vi "ConfigureSequencerElement.vi"(4 "error in (no error)":errorcluster, 5 "Sequencer Element":i16=1, 6 "Sequencer Item":T1={"Entry Length"=16384, "Repetition Count"=1, "Infinite Repetitions"=FALSE, "Channels"=[{"Analog Waveform"="SINE", "Amplitude [V]"=2.0, "Offset [V]"=0.0}, {"Analog Waveform"="SINE", "Amplitude [V]"=2.0, "Offset [V]"=0.0}], "Digital Waveform"=""} {"Repetition Count" min=1}, 7 "VISA resource name":refnum<visa-resource-name>) -> (0 "error out":errorcluster, 3 "VISA resource name out":refnum<visa-resource-name>)   [LabVIEW 2020, in "Active Technologies AWG3000.lvlib"]
uses:
  Active Technologies AWG3000.lvlib
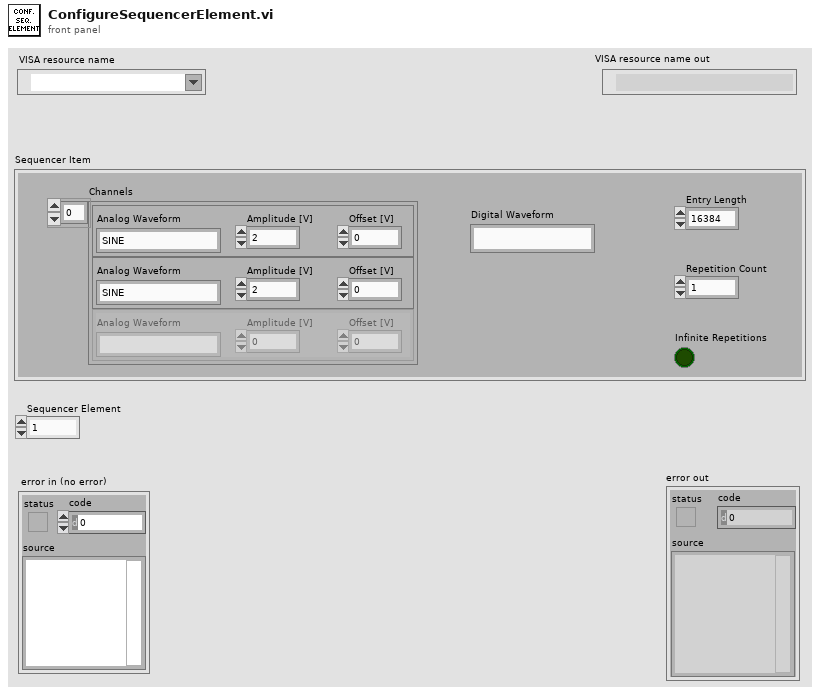
[diagram p1: front panel]
types:
  T1 = cluster{"Entry Length":i32, "Repetition Count":i32, "Infinite Repetitions":bool, "Channels":cluster{"Analog Waveform":string, "Amplitude [V]":dbl, "Offset [V]":dbl}[], "Digital Waveform":string}
  T2 = cluster{"Analog Waveform":string, "Amplitude [V]":dbl, "Offset [V]":dbl}[]
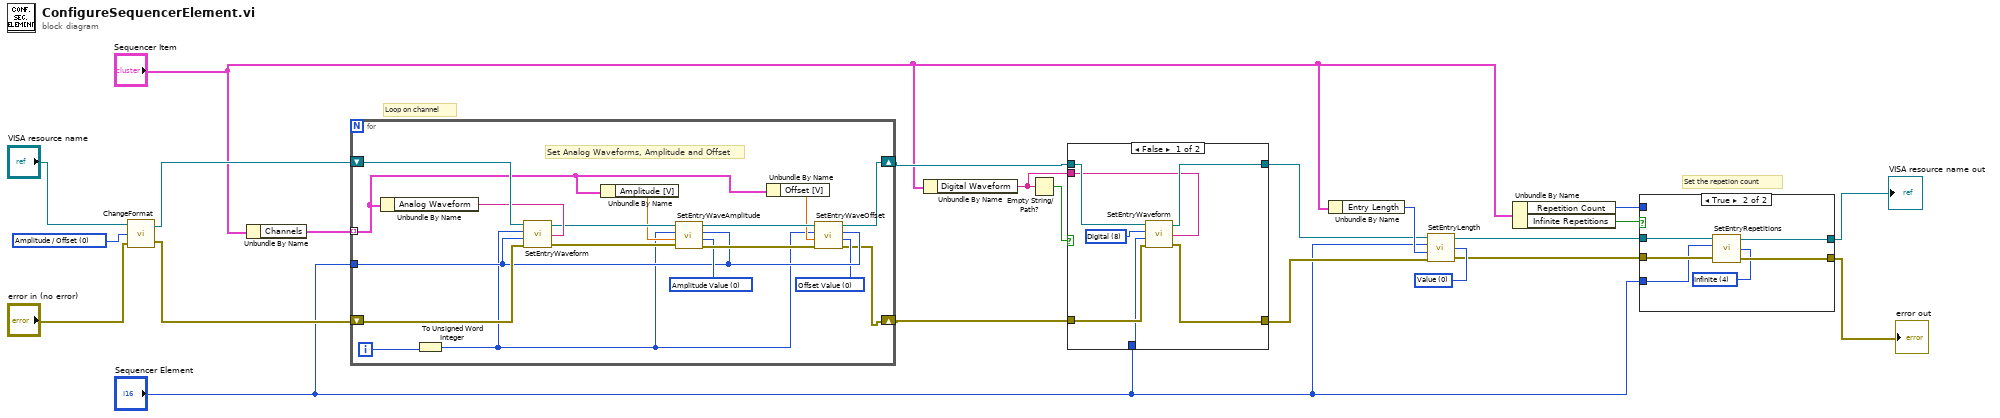
[diagram p0: block diagram]
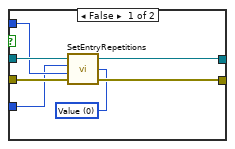
[diagram p3: hidden frame]
diagram:
  w9 = u8 0 items=["Amplitude / Offset", "Voltage High / Voltage Low"] ("Format")
  w20 = u16 0 items=["Value", "Default", "Minimum", "Maximum"] ("Entry Length Options")
  # "Set the repetion count"
  # "Loop on channel"
  n1 = call "ChangeFormat.vi"("error in (no error)"="error in (no error)", "Format"=w9, "VISA resource name"="VISA resource name") -> ("error out"=w10:errorcluster, "VISA resource name out"=w12:refnum<visa-resource-name>)
  n2 = Unbundle By Name("Sequencer Item") -> ("Channels"=w22:T2)
  n3 = for {
    tunnel: w22 -> [w26] mode=indexing
    tunnel: "Sequencer Element" -> [w29]
    shift-right: [w25] -> w6
    shift-left: w12 -> [w39]
    shift-right: [w24] -> w5
    shift-left: w10 -> [w38]
    i -> [w27]
    w28 = u16 0 items=["Offset Value", "Default", "Minimum", "Maximum"] ("Offset Options")
    w31 = u16 0 items=["Amplitude Value", "Default", "Minimum", "Maximum"] ("Amplitude Options")
    # "Set Analog Waveforms, Amplitude and Offset"
    n4 = Unbundle By Name(w26) -> ("Analog Waveform"=w37:string)
    n5 = To Unsigned Word Integer(number=w27) -> (unsigned 16bit integer=w23:u16)
    n6 = call "SetEntryWaveform.vi"("Waveform Name"=w37, "error in (no error)"=w38, "Element"=w29, "Channel"=w23, "VISA resource name"=w39) -> ("error out"=w35:errorcluster, "VISA resource name out"=w36:refnum<visa-resource-name>)
    n7 = Unbundle By Name(w26) -> ("Amplitude [V]"=w34:dbl)
    n8 = call "SetEntryWaveAmplitude.vi"("Amplitude Options"=w31, "Element"=w29, "error in (no error)"=w35, "Amplitude (Vpp)"=w34, "Channel"=w23, "VISA resource name"=w36) -> ("error out"=w32:errorcluster, "VISA resource name out"=w33:refnum<visa-resource-name>)
    n9 = Unbundle By Name(w26) -> ("Offset [V]"=w30:dbl)
    n10 = call "SetEntryWaveOffset.vi"("Offset Options"=w28, "Element"=w29, "error in (no error)"=w32, "Offset (V)"=w30, "Channel"=w23, "VISA resource name"=w33) -> ("error out"=w24:errorcluster, "VISA resource name out"=w25:refnum<visa-resource-name>)
  }
  n11 = Unbundle By Name("Sequencer Item") -> ("Digital Waveform"=w7:string)
  n12 = Empty String/Path?(string/path=w7) -> (empty?=w8:bool)
  n13 = case shown="False" w8 {
    tunnel: w6 -> [w46 w48]
    tunnel: [w45 w48] -> w4
    tunnel: [w43 w47] -> w3
    tunnel: w5 -> [w44 w47]
    tunnel: "Sequencer Element" -> [w42 _]
    tunnel: w7 -> [w41 _]
    frame False {
      w40 = u16 8 items=["Channel 1", "Channel 2", "Channel 3", "Channel 4", "Channel 5", "Channel 6", "Channel 7", "Channel 8", "Digital"] ("Channel")
      n14 = call "SetEntryWaveform.vi"("Waveform Name"=w41, "error in (no error)"=w44, "Element"=w42, "Channel"=w40, "VISA resource name"=w46) -> ("error out"=w43:errorcluster, "VISA resource name out"=w45:refnum<visa-resource-name>)
    }
    frame True {
    }
  }
  n15 = Unbundle By Name("Sequencer Item") -> ("Entry Length"=w21:i32)
  n16 = call "SetEntryLength.vi"("Entry Length Options"=w20, "error in (no error)"=w3, "Length (N)"=w21, "Element"="Sequencer Element", "VISA resource name"=w4) -> ("error out"=w18:errorcluster, "VISA resource name out"=w19:refnum<visa-resource-name>)
  n17 = Unbundle By Name("Sequencer Item") -> ("Repetition Count"=w16:i32, "Infinite Repetitions"=w17:bool)
  n18 = case shown="True" w17 {
    tunnel: w19 -> [w55 w61]
    tunnel: w18 -> [w54 w60]
    tunnel: w16 -> [w53 _]
    tunnel: [w52 w59] -> w15
    tunnel: [w51 w58] -> w14
    tunnel: "Sequencer Element" -> [w50 w56]
    frame False {
      w49 = u16 0 items=["Value", "Default", "Minimum", "Maximum"] ("Entry Repetitions Options")
      n19 = call "SetEntryRepetitions.vi"("Entry Repetitions Options"=w49, "error in (no error)"=w54, "Entry Repetitions (N)"=w53, "Element"=w50, "VISA resource name"=w55) -> ("error out"=w51:errorcluster, "VISA resource name out"=w52:refnum<visa-resource-name>)
    }
    frame True {
      w57 = u16 4 items=["Value", "Default", "Minimum", "Maximum", "Infinite"] ("Entry Repetitions Options")
      n20 = call "SetEntryRepetitions.vi"("Entry Repetitions Options"=w57, "error in (no error)"=w60, "Element"=w56, "VISA resource name"=w61) -> ("error out"=w58:errorcluster, "VISA resource name out"=w59:refnum<visa-resource-name>)  [unwired: 1 in]
    }
  }
  "VISA resource name out" <- w15
  "error out" <- w14
